vi "readPulsatorPositionAndSpeed.vi"(8 "comms":T2, 10 "message scheduler":refnum<class "message scheduler.lvclass">, 11 "Queues":T1) -> ()   [LabVIEW 2018]
uses:
  type defs/comms loop data.ctl
  ICL-LabVIEW_General/Incident logger/Incident logger.lvclass
  <vilib>/Modbus/master/Modbus Master.lvclass
  type defs/Queues.ctl
  ICL-LabVIEW_General/Message Scheduler/message scheduler.lvclass
  ICL-LabVIEW_General/Pulser Controller/AKD MODBUS commands/get position.vi
  ICL-LabVIEW_General/Pulser Controller/AKD MODBUS commands/get velocity.vi
  supporting VIs/polymorphic VIs/enqueue for user interface.vi
  ICL-LabVIEW_General/Pulser Controller/Pulser controller commands library.lvlib
  ICL-LabVIEW_General/Message Scheduler/scheduled message/scheduled message.lvclass
panel:
  out "pulsator state":cluster{"poition":i32, "velocity":i32}
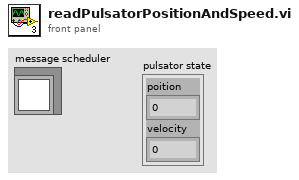
[diagram p1: front panel]
types:
  T1 = typedef "Queues.ctl" = cluster{"messageHandler":refnum<queue>, "comms":refnum<queue>, "dataStream":refnum<queue>, "dataProcessor":refnum<queue>, "fileIO":refnum<queue>, "userInterface":refnum<queue>, "errors":refnum<queue>, "customCompressor":refnum<queue>}
  T2 = typedef "comms loop data.ctl" = cluster{"params":cluster{"commandStream":cluster{"reader name":string, "writer name":string, "stream buffer size":i32}, "errorStream":cluster{"reader name":string, "writer name":string, "stream buffer size":i32}, "RT IP address":string, "pulserControllerIP":string}, "vars":cluster{"commandStream":refnum<k21>, "Incident logger":refnum<class "Incident logger.lvclass">, "check error scheduled message":u32, "errorStream":refnum<k21>, "watchdogScheduleID":u32, "pulsator":cluster{"pulser connection":refnum<class "Modbus Master.lvclass">, "pulserConnected":bool, "pulsatorScheduleID":u32, "pulserRunning":bool}}}
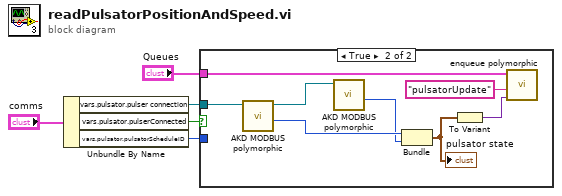
[diagram p0: block diagram]
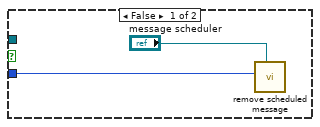
[diagram p2: hidden frame]
diagram:
  n1 = Unbundle By Name("comms") -> ("vars.pulsator.pulser connection"=w2:refnum<class "Modbus Master.lvclass">, "vars.pulsator.pulserConnected"=w4:bool, "vars.pulsator.pulsatorScheduleID"=w3:u32)
  n2 = case shown="True" w4 {
    tunnel: w3 -> [w6 _]
    tunnel: w2 -> [_ w15]
    tunnel: "Queues" -> [_ w13]
    frame False {
      n3 = call "remove scheduled message.vi"("message scheduler"="message scheduler", "schedule ID"=w6) -> ()  [unwired: 9 in, 1 out]
    }
    frame True {
      n4 = call-poly "AKD MODBUS polymorphic.vi"("Modbus Master in"=w15) -> ("poition"=w11:i32, "Modbus Master out"=w14:refnum<class "Modbus Master.lvclass">)  [unwired: 8 in, 1 out]
      n5 = call-poly "AKD MODBUS polymorphic.vi"("Modbus Master in"=w14) -> ("velocity"=w10:i32)  [unwired: 8 in, 2 out]
      n6 = Bundle("poition"=w11, "velocity"=w10) -> (w9:cluster{"poition":i32, "velocity":i32})  [unwired: 1 in]
      "pulsator state" <- w9
      n7 = To Variant(anything=w9) -> (Variant=w8:variant)
      n8 = call-poly "enqueue polymorphic.vi"("data"=w8, "message"="pulsatorUpdate", "Queues"=w13) -> ()  [unwired: 8 in, 1 out]
    }
  }
